vi "Module Pre-Loop Init.vi"(8 "error in (no error)":errorcluster, 11 "Top Level VI Ref in":refnum<vi>) -> (0 "error out":errorcluster, 3 "User Event Stop Ref":refnum<event-registration>)   [LabVIEW 2018, in "Error Handler.lvlib"]
doc: "This subVI completes all initialization for communications and user events at the beginning of the top-level VI."
uses:
  Error Handler.lvlib
  Private Controls/Module Data.ctl
  Private Controls/Module Action.ctl
  Private Controls/Queue Comms FGV Action.ctl
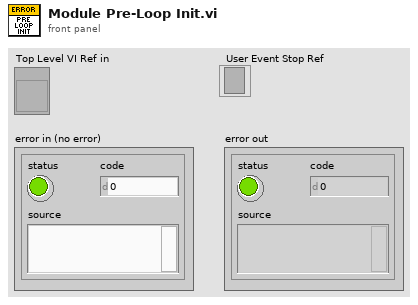
[diagram p1: front panel]
types:
  T1 = typedef "Error Handler.lvlib/Queue Comms FGV Action.ctl" = enum16{"Get", "Set", "Release"}
  T2 = typedef "Error Handler.lvlib/Module Data.ctl" = cluster{"Data":variant, "Action":T3}
  T3 = typedef "Error Handler.lvlib/Module Action.ctl" = enum8{"Init", "Exit", "Controller Error", "UI1 Error", "UI2 Error", "UI3 Error", "File IO Error", "cRIO Error", "Calibration Error"}
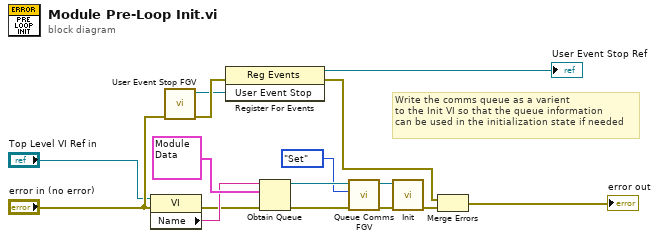
[diagram p0: block diagram]
diagram:
  # "Write the comms queue as a varient\nto the Init VI so that the queue information\ncan be used in the initialization state if needed"
  n1 = property class="VI"(reference="Top Level VI Ref in", error in="error in (no error)") -> (error out=w5:errorcluster, "Name"=w6:string)  [unwired: 1 out]
  n2 = call "User Event Stop FGV.vi"("error in (no error)"="error in (no error)") -> ("error out"=w2:errorcluster, "User Event Stop"=w1:refnum<user-event>)  [unwired: 9 in]
  n3 = register-events(error in=w2, w1) -> (reference out=→"User Event Stop Ref":refnum<event-registration>, error out=w14:errorcluster)  [unwired: 1 in]
  n4 = Obtain Queue(name (unnamed)=w6, element data type=T2 {"Data"=variant, "Action"=enum."Init"} ("Module Data"), error in (no error)=w5) -> (queue out=w9:refnum<queue>, error out=w10:errorcluster)  [unwired: 2 in, 1 out]
  n5 = call "Queue Comms FGV.vi"("error in (no error)"=w10, "Action (Get)"=Queue_Comms_FGV_Action."Set", "Queue in"=w9) -> ("error out"=w11:errorcluster, "Queue out"=w12:refnum<queue>)  [unwired: 7 in]
  n6 = call "Init.vi"("error in (no error)"=w11, "Data"=w12) -> ("error out"=w13:errorcluster)  [unwired: 9 in]
  n7 = Merge Errors(w14, w13) -> (→"error out":errorcluster)
